vi "Sub_GuidanceMatrix.vi"(0 "距离":dbl=1.0 format="%#_13g") -> (14 "平移采样点信息":dbl[][](array[numeric]))   [LabVIEW 2018]
uses:
  <vilib>/Utility/file.llb/Read Delimited Spreadsheet (DBL).vi
panel:
  out "阵列坐标":dbl[][](array[numeric])
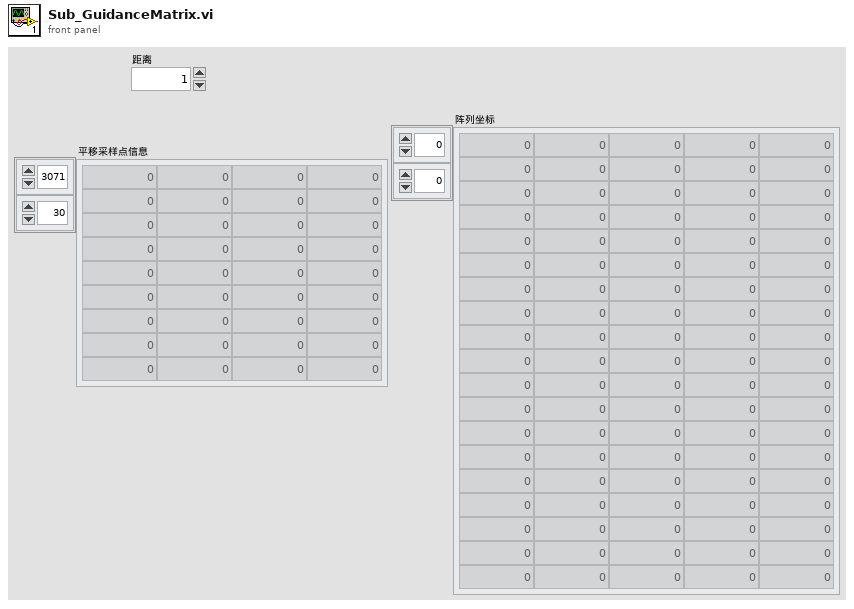
[diagram p1: front panel]
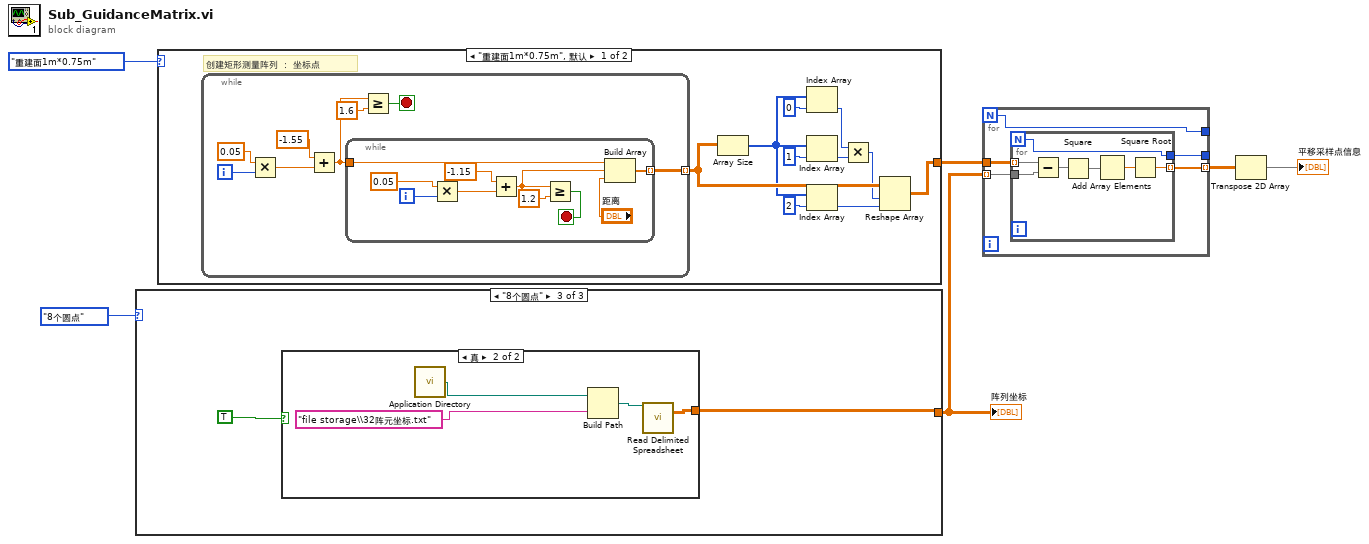
[diagram p0: block diagram]
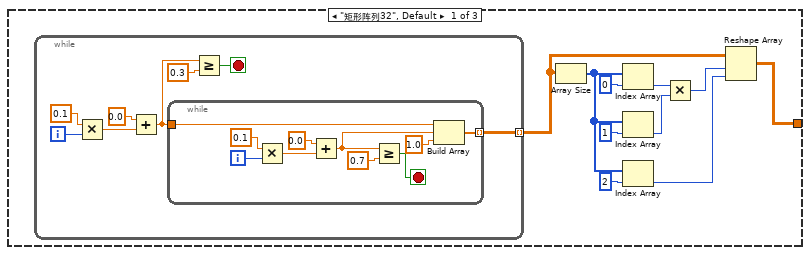
[diagram p2: hidden frame]
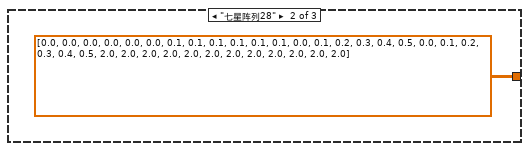
[diagram p3: hidden frame]
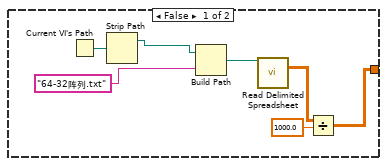
[diagram p4: hidden frame]
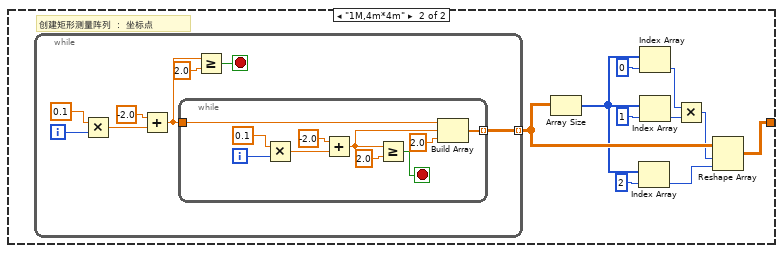
[diagram p5: hidden frame]
diagram:
  n1 = case shown="\"8个圆点\"" enum16{"矩形阵列32", "8个圆点", "七星阵列28", ""}."8个圆点" ("操作(0:open)") {
    tunnel: [w7 dbl[][] [[0.0, 0.0, 0.0, 0.0, 0.0, 0.0, 0.1, 0.1, 0.1, 0.1, 0.1, 0.1], [0.0, 0.1, 0.2, 0.3, 0.4, 0.5, 0.0, 0.1, 0.2, 0.3, 0.4, 0.5], [2.0, 2.0, 2.0, 2.0, 2.0, 2.0, 2.0, 2.0, 2.0, 2.0, 2.0, 2.0]] w37] -> w3
    frame "矩形阵列32", Default {
      n2 = while {
        tunnel: [w17] -> w8 mode=indexing
        i -> [w24]
        stop <- w20 stop-if-true
        n3 = Multiply(x=0.1, y=w24) -> (x*y=w22:dbl)
        n4 = Add(x=0.0, y=w22) -> (x+y=w18:dbl)
        n5 = while {
          tunnel: [w26] -> w17 mode=indexing
          tunnel: w18 -> [w28]
          i -> [w29]
          stop <- w31 stop-if-true
          n6 = Multiply(x=0.1, y=w29) -> (x*y=w33:dbl)
          n7 = Add(x=0.0, y=w33) -> (x+y=w27:dbl)
          n8 = Greater Or Equal?(x=w27, y=0.7) -> (x >= y?=w31:bool)
          n9 = Build Array(w28, w27, 1.0 ("元素")) -> (w26:dbl[])
        }
        n10 = Greater Or Equal?(x=w18, y=0.3) -> (x >= y?=w20:bool)
      }
      n11 = Array Size(array=w8) -> (size(s)=w13:i32[])
      n12 = Index Array(array=w13, index=0 ("索引")) -> (element=w12:i32)
      n13 = Index Array(array=w13, index=1 ("索引")) -> (element=w11:i32)
      n14 = Index Array(array=w13, index=2 ("索引")) -> (element=w9:i32)
      n15 = Multiply(x=w12, y=w11) -> (x*y=w10:i32)
      n16 = Reshape Array(w8, w10, w9) -> (w7:dbl[][])
    }
    frame "七星阵列28" {
    }
    frame "8个圆点" {
      n17 = case shown="真" TRUE {
        tunnel: [w40 w47] -> w37
        frame False {
          n18 = Current VI's Path() -> (path=w42:path)
          n19 = Strip Path(path=w42) -> (stripped path=w38:path)  [unwired: 1 out]
          n20 = Build Path(base path=w38, name or relative path="64-32阵列.txt" ("名称或相对路径")) -> (appended path=w43:path)
          n21 = call-poly <vilib>:"Read Delimited Spreadsheet.vi"("file path (dialog if empty)"=w43) -> ("all rows"=w41:dbl[][])  [unwired: 9 in, 5 out]
          n22 = Divide(x=w41, y=1000.0) -> (x/y=w40:dbl[][])
        }
        frame True {
          n23 = call <vilib>:"Application Directory.vi"() -> ("Application Directory"=w45:path)
          n24 = Build Path(base path=w45, name or relative path="file storage\\32阵元坐标.txt" ("名称或相对路径")) -> (appended path=w48:path)
          n25 = call-poly <vilib>:"Read Delimited Spreadsheet.vi"("file path (dialog if empty)"=w48) -> ("all rows"=w47:dbl[][])  [unwired: 9 in, 5 out]
        }
      }
    }
  }
  "阵列坐标" <- w3
  n26 = case shown="\"重建面1m*0.75m\", 默认" enum16{"重建面1m*0.75m", "1M,4m*4m", ""}."重建面1m*0.75m" ("操作(0:open)") {
    tunnel: [w49 w77] -> w5
    frame "重建面1m*0.75m", Default {
      # "创建矩形测量阵列 ： 坐标点"
      n27 = while {
        tunnel: [w59] -> w58 mode=indexing
        i -> [w66]
        stop <- w62 stop-if-true
        n28 = Multiply(x=0.05, y=w66) -> (x*y=w64:dbl)
        n29 = Add(x=-1.55, y=w64) -> (x+y=w60:dbl)
        n30 = while {
          tunnel: [w68] -> w59 mode=indexing
          tunnel: w60 -> [w70]
          i -> [w71]
          stop <- w73 stop-if-true
          n31 = Multiply(x=0.05, y=w71) -> (x*y=w75:dbl)
          n32 = Add(x=-1.15, y=w75) -> (x+y=w69:dbl)
          n33 = Greater Or Equal?(x=w69, y=1.2) -> (x >= y?=w73:bool)
          n34 = Build Array(w70, w69, "距离") -> (w68:dbl[])
        }
        n35 = Greater Or Equal?(x=w60, y=1.6) -> (x >= y?=w62:bool)
      }
      n36 = Array Size(array=w58) -> (size(s)=w54:i32[])
      n37 = Index Array(array=w54, index=0 ("索引")) -> (element=w53:i32)
      n38 = Index Array(array=w54, index=1 ("索引")) -> (element=w52:i32)
      n39 = Index Array(array=w54, index=2 ("索引")) -> (element=w50:i32)
      n40 = Multiply(x=w53, y=w52) -> (x*y=w51:i32)
      n41 = Reshape Array(w58, w51, w50) -> (w49:dbl[][])
    }
    frame "1M,4m*4m" {
      # "创建矩形测量阵列 ： 坐标点"
      n42 = while {
        tunnel: [w87] -> w86 mode=indexing
        i -> [w94]
        stop <- w90 stop-if-true
        n43 = Multiply(x=0.1, y=w94) -> (x*y=w92:dbl)
        n44 = Add(x=-2.0, y=w92) -> (x+y=w88:dbl)
        n45 = while {
          tunnel: [w96] -> w87 mode=indexing
          tunnel: w88 -> [w98]
          i -> [w99]
          stop <- w101 stop-if-true
          n46 = Multiply(x=0.1, y=w99) -> (x*y=w103:dbl)
          n47 = Add(x=-2.0, y=w103) -> (x+y=w97:dbl)
          n48 = Greater Or Equal?(x=w97, y=2.0) -> (x >= y?=w101:bool)
          n49 = Build Array(w98, w97, 2.0) -> (w96:dbl[])
        }
        n50 = Greater Or Equal?(x=w88, y=2.0) -> (x >= y?=w90:bool)
      }
      n51 = Array Size(array=w86) -> (size(s)=w82:i32[])
      n52 = Index Array(array=w82, index=2 ("索引")) -> (element=w78:i32)
      n53 = Index Array(array=w82, index=0 ("索引")) -> (element=w81:i32)
      n54 = Index Array(array=w82, index=1 ("索引")) -> (element=w80:i32)
      n55 = Multiply(x=w81, y=w80) -> (x*y=w79:i32)
      n56 = Reshape Array(w86, w79, w78) -> (w77:dbl[][])
    }
  }
  n57 = for {
    N -> [w105]
    tunnel: w3 -> [w109] mode=indexing
    tunnel: w5 -> [w108]
    tunnel: [w107] -> w4 mode=indexing
    tunnel: [w106] -> _
    tunnel: [w105] -> _
    n58 = for {
      N -> [w110]
      tunnel: w109 -> [w115]
      tunnel: w108 -> [w116] mode=indexing
      tunnel: [w111] -> w107 mode=indexing
      tunnel: [w110] -> w106
      n59 = Subtract(x=w116, y=w115) -> (x-y=w114:dbl[])
      n60 = Square(x=w114) -> (x^2=w113:dbl[])
      n61 = Add Array Elements(numeric array=w113) -> (sum=w112:dbl)
      n62 = Square Root(x=w112) -> (sqrt(x)=w111:dbl)
    }
  }
  n63 = Transpose 2D Array(2D array=w4) -> (transposed array=→"平移采样点信息":dbl[][])
